vi "Lvi Read U32Data1D.vi"(7 "OnlyReadAvailable":bool, 8 "error in (no error)":errorcluster, 9 "timeout":dbl, 10 "TaskRef":i32, 11 "DataBufSize":u32) -> (0 "error out":errorcluster, 1 "DataBuf":u32[](array[numeric]), 2 "TaskRef out":i32, 3 "DataBufSize out":u32, 5 "function return":i32)   [LabVIEW 2016, in "DtLvLink.lvlib"]
doc: "Calls directly into the entry points of the DLL of the Data Acq SDK to return a one-dimensional array of unsigned, 32-bit integers representing the data points from the specified task."
uses:
  <userlib>/LV-Link3/DtLvLink.lvlib
  <userlib>/LV-Link3/DtLvLink_32.dll
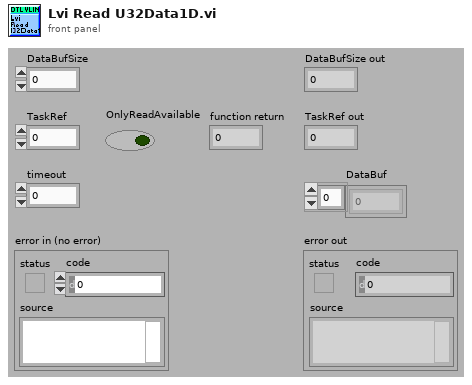
[diagram p1: front panel]
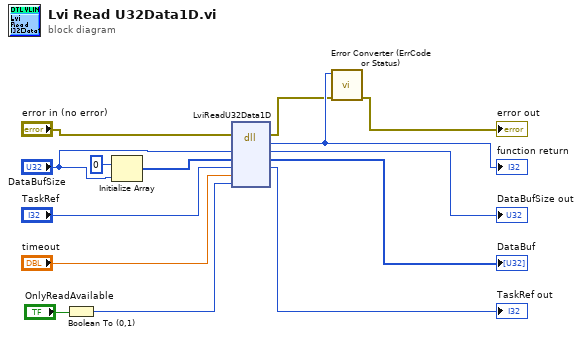
[diagram p0: block diagram]
diagram:
  n1 = Boolean To (0,1)(Boolean="OnlyReadAvailable") -> (0, 1=w1:i16)
  n2 = Initialize Array(u32 0 ("element"), "DataBufSize") -> (w11:u32[])
  n3 = dll-call lib="C:/Program Files (x86)/National Instruments/LabVIEW 2016/user.lib/LV-Link3/DtLvLink_32.*" fn="LviReadU32Data1D"(error in="error in (no error)", "DataBufSize"="DataBufSize", "DataBuf"=w11, "TaskRef"="TaskRef", "timeout"="timeout", "OnlyReadAvailable"=w1) -> (error out=w4:errorcluster, "return type"=w14:i32, "DataBufSize"=→"DataBufSize out":u32, "DataBuf"=→"DataBuf":u32[], "TaskRef"=→"TaskRef out":i32)  [unwired: 4 in, 1 out]
  "function return" <- w14
  n4 = call <userlib>:"Error Converter (ErrCode or Status).vi"("error in (no error)"=w4, "error code"=w14) -> ("error out"=→"error out":errorcluster)  [unwired: 9 in]
